vi "E2 Lookup Table Get Value.vi"(10 "Fractional Input":dbl, 11 "Array of XY Data Points":cluster{"X":dbl, "Y":dbl}[](array[cluster])) -> (2 "Interpolated Output":dbl)   [LabVIEW 2015]
panel:
  # "OUTPUTS"
  # "INPUTS"
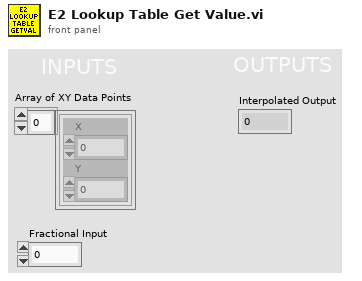
[diagram p1: front panel]
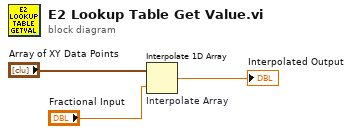
[diagram p0: block diagram]
diagram:
  n1 = Interpolate 1D Array "Interpolate Array"(1:"Fractional Input", 2:"Array of XY Data Points") -> (0:→"Interpolated Output":dbl)
